vi "Refresh Tag Exchange Tables.vi"(6 "Tag Exchange Tab References":T1, 7 "Filter":string, 8 "error in (no error)":errorcluster, 10 "engine":refnum<data-value>, 11 "E2E editor node in":refnum<data-value>) -> (0 "error out":errorcluster, 2 "engine out":refnum<data-value>, 3 "E2E editor node out":refnum<data-value>)   [LabVIEW 2015, in "E2E Tag Exchange editor node.lvclass"]
uses:
  E2E Tag Exchange editor node.lvclass
  Tag Exchange Tab References.ctl
  <vilib>/NI/DCAF/Tag Editor Core/Configuration Editor/Classes/Engine Parent/Engine Parent Editor Node.lvclass
  <vilib>/NI/Tag Bus/tag/tag descriptor.lvclass/tag descriptor.ctl
  Apply Filter_2D.vi
  Apply Filter_1D.vi
  <vilib>/NI/Tag Bus/tag/tag descriptor.lvclass
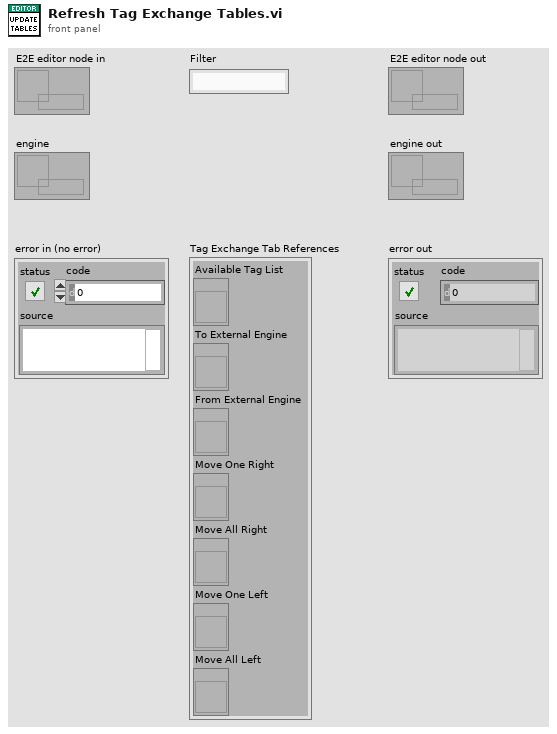
[diagram p1: front panel]
types:
  T1 = typedef "E2E Tag Exchange editor node.lvclass/Tag Exchange Tab References.ctl" = cluster{"Available Tag List":refnum<vi>, "To External Engine":refnum<vi>, "From External Engine":refnum<vi>, "Move One Right":refnum<vi>, "Move All Right":refnum<vi>, "Move One Left":refnum<vi>, "Move All Left":refnum<vi>}
  T2 = typedef "tag bus.lvlib/tag descriptor.lvclass/Data Type.ctl" = enum16{"Double", "Single", "I64", "I32", "I16", "I8", "U64", "U32", "U16", "U8", "Boolean", "String", "Array of Double", "Array of Single", "Array of I64", "Array of I32", "Array of I16", "Array of I8", "Array of U64", "Array of U32", "Array of U16", "Array of U8", "Array of Boolean", "Array of String"}
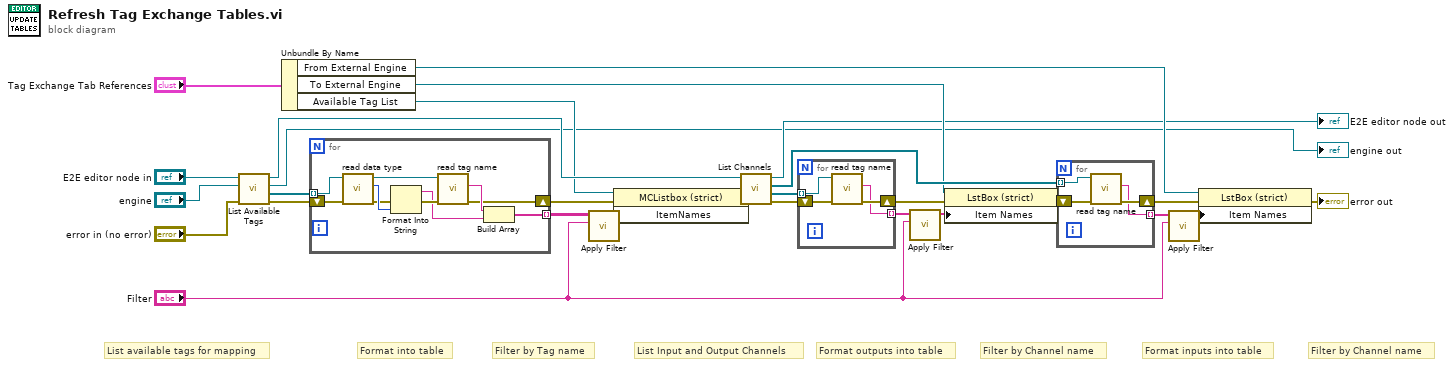
[diagram p0: block diagram]
diagram:
  # "Filter by Channel name"
  # "Format inputs into table"
  # "Filter by Channel name"
  # "Format outputs into table"
  # "List Input and Output Channels"
  # "Filter by Tag name"
  # "Format into table"
  # "List available tags for mapping"
  n1 = call "List Available Tags.vi"("error in (no error)"="error in (no error)", "engine"="engine", "E2E editor node in"="E2E editor node in") -> ("error out"=w6:errorcluster, "Available Tags"=w7:refnum<class "tag descriptor.lvclass">[], "engine out"=→"engine out":refnum<data-value>, "E2E editor node out"=w15:refnum<data-value>)  [unwired: 5 in]
  n2 = Unbundle By Name("Tag Exchange Tab References") -> ("From External Engine"=w26:refnum<vi>, "To External Engine"=w20:refnum<vi>, "Available Tag List"=w12:refnum<vi>)
  n3 = for {
    tunnel: w7 -> [w34] mode=indexing
    shift-right: [w29] -> w11
    shift-left: w6 -> [w35]
    tunnel: [w30] -> w9 mode=indexing
    n4 = call <vilib>:"read data type.vi"("error in"=w35, "system tag in"=w34) -> ("error out"=w37:errorcluster, "data type"=w38:T2, "system tag out"=w33:refnum<class "tag descriptor.lvclass">)  [unwired: 7 in]
    n5 = Format Into String(error in=w37, w38) -> (resulting string=w32:string, error out=w36:errorcluster)  [unwired: 2 in]
    n6 = call <vilib>:"read tag name.vi"("error in"=w36, "system tag in"=w33) -> ("error out"=w29:errorcluster, "name"=w31:string)  [unwired: 7 in, 1 out]
    n7 = Build Array(w31, w32) -> (w30:string[])
  }
  n8 = call-poly "Apply Filter.vi"("Filter"="Filter", "Items to Filter"=w9) -> ("Filtered Items"=w13:string[][])  [unwired: 9 in]
  n9 = property class="MCListbox (strict)"(reference=w12, error in=w11, "ItemNames"=w13) -> (error out=w14:errorcluster)  [unwired: 1 out]
  n10 = call "List Channels.vi"("error in (no error)"=w14, "E2E editor node in"=w15) -> ("error out"=w16:errorcluster, "Output Channels"=w17:refnum<class "TBM channel.lvclass">[], "Input Channels"=w23:refnum<class "TBM channel.lvclass">[], "E2E editor node out"=→"E2E editor node out":refnum<data-value>)  [unwired: 6 in]
  n11 = for {
    tunnel: w17 -> [w42] mode=indexing
    shift-right: [w40] -> w19
    shift-left: w16 -> [w41]
    tunnel: [w39] -> w18 mode=indexing
    n12 = call <vilib>:"read tag name.vi"("error in"=w41, "system tag in"=w42) -> ("error out"=w40:errorcluster, "name"=w39:string)  [unwired: 7 in, 1 out]
  }
  n13 = call-poly "Apply Filter.vi"("Filter"="Filter", "Items to Filter"=w18) -> ("Filtered Items"=w21:string[])  [unwired: 9 in]
  n14 = property class="LstBox (strict)"(reference=w20, error in=w19, "Item Names"=w21) -> (error out=w22:errorcluster)  [unwired: 1 out]
  n15 = for {
    shift-right: [w45] -> w24
    shift-left: w22 -> [w46]
    tunnel: w23 -> [w44] mode=indexing
    tunnel: [w43] -> w25 mode=indexing
    n16 = call <vilib>:"read tag name.vi"("error in"=w46, "system tag in"=w44) -> ("error out"=w45:errorcluster, "name"=w43:string)  [unwired: 7 in, 1 out]
  }
  n17 = call-poly "Apply Filter.vi"("Filter"="Filter", "Items to Filter"=w25) -> ("Filtered Items"=w28:string[])  [unwired: 9 in]
  n18 = property class="LstBox (strict)"(reference=w26, error in=w24, "Item Names"=w28) -> (error out=→"error out":errorcluster)  [unwired: 1 out]
